vi "Draw Action Diagram.vi"(7 "Diagram Ref":refnum<vi>, 10 "Actions":T1) -> (2 "Action Diagram":picture)   [LabVIEW 2022 SP3, in "FlexBlocks Support.lvlib"]
uses:
  FlexBlocks Support.lvlib
  Action Selections.ctl
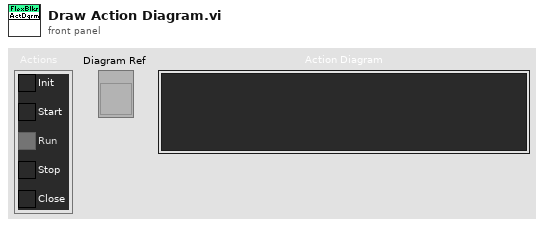
[diagram p1: front panel]
types:
  T1 = typedef "FlexBlocks Support.lvlib/Action Selections.ctl" = cluster{"Init":bool, "Start":bool, "Run":bool, "Stop":bool, "Close":bool}
  T2 = cluster{"left":i16, "top":i16, "right":i16, "bottom":i16}
  T3 = typedef "FlexBlocks Support.lvlib/Action Diagram Sizing.ctl" = cluster{"Start X":i32, "Node Spacing":i32, "Node Height":i32, "Node Center Offset":i32, "Terminus Spacing":i32, "Node Width":i32, "Total Width":i32, "Top":i32, "Inner Top":i32, "Outer Top":i32, "Line left":i32, "Line top":i32, "Line right":i32}
  T4 = cluster{"horizontal":enum16{"left", "center", "right"}, "vertical":enum16{"top", "center", "bottom"}}
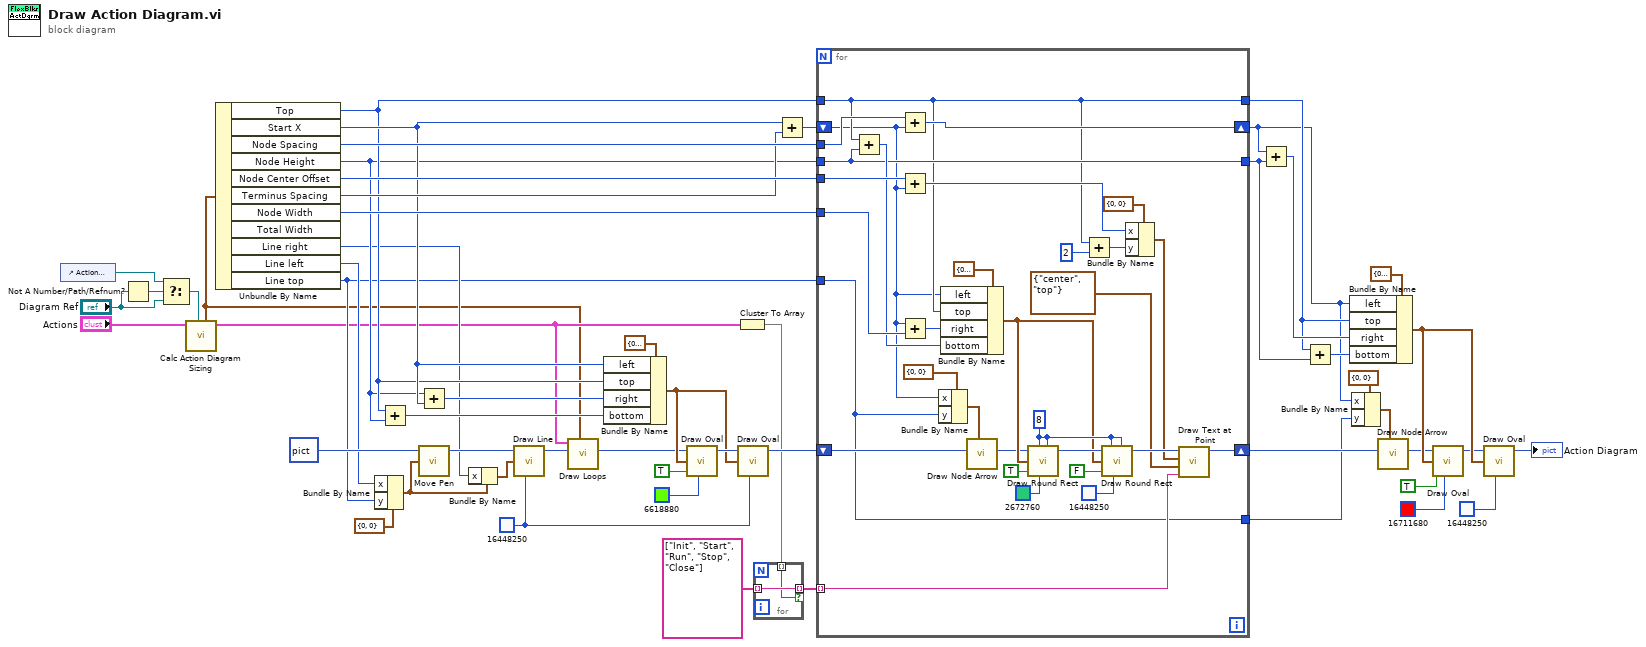
[diagram p0: block diagram]
diagram:
  w16 = u32 16448250 ("color(black)")
  n1 = control-ref of="Action Diagram"() -> (w25:refnum<vi>)
  n2 = Not A Number/Path/Refnum?(number/path/refnum="Diagram Ref") -> (NaN/Path/Refnum?=w26:bool)
  n3 = Select(t=w25, s=w26, f="Diagram Ref") -> (s? t:f=w23:refnum<vi>)
  n4 = call "Calc Action Diagram Sizing.vi"("Diagram Ref"=w23, "Actions In"="Actions") -> ("Actions"=w2:T1, "Action Diagram Sizing"=w1:T3)  [unwired: 8 in]
  n5 = Unbundle By Name(w1) -> ("Top"=w19:i32, "Start X"=w20:i32, "Node Spacing"=w36:i32, "Node Height"=w18:i32, "Node Center Offset"=w35:i32, "Terminus Spacing"=w32:i32, "Node Width"=w33:i32, "Line right"=w12:i32, "Line left"=w13:i32, "Line top"=w11:i32)  [unwired: 1 out]
  n6 = Bundle By Name(cluster=cluster{"x":i16, "y":i16} {"x"=0, "y"=0} ("new position"), "x"=w13, "y"=w11) -> (w15:cluster{"x":i16, "y":i16})
  n7 = Add(x=w19, y=w18) -> (x+y=w46:i32)
  n8 = Add(x=w18, y=w20) -> (x+y=w34:i32)
  n9 = call <vilib>:"Move Pen.vi"("new position"=w15, "picture"=picture data[5B] ("Action Diagram")) -> ("new picture"=w17:picture)  [unwired: 3 in]
  n10 = Bundle By Name(cluster=w15, "x"=w12) -> (w14:cluster{"x":i16, "y":i16})
  n11 = call <vilib>:"Draw Line.vi"("picture"=w17, "end point"=w14, "color(black)"=w16) -> ("new picture"=w4:picture)  [unwired: 6 in]
  n12 = call "Draw Loops.vi"("Action Diagram Sizing"=w1, "Action Diagram In"=w4, "Actions"=w2) -> ("Action Diagram"=w3:picture)  [unwired: 8 in]
  n13 = Bundle By Name(cluster=T2 {"left"=0, "top"=0, "right"=0, "bottom"=0} ("rect"), "left"=w20, "top"=w19, "right"=w34, "bottom"=w46) -> (w47:T2)
  n14 = call <vilib>:"Draw Oval.vi"("picture"=w3, "rect"=w47, "fill?(F)"=TRUE, "color(black)"=u32 6618880) -> ("new picture"=w49:picture)  [unwired: 5 in]
  n15 = Cluster To Array(cluster=w2) -> (array=w37:bool[])
  n16 = call <vilib>:"Draw Oval.vi"("picture"=w49, "rect"=w47, "color(black)"=w16) -> ("new picture"=w48:picture)  [unwired: 6 in]
  n17 = for {
    tunnel: string[] ["Init", "Start", "Run", "Stop", "Close"] -> [w56] mode=indexing
    tunnel: [w56] -> w53 mode=indexing if=w55
    tunnel: w37 -> [w55] mode=indexing
  }
  n18 = Add(x=w20, y=w32) -> (x+y=w31:i32)
  n19 = for {
    shift-right: [w79] -> w10
    shift-left: w48 -> [w61]
    tunnel: w53 -> [w78] mode=indexing
    tunnel: w19 -> [w63]
    tunnel: w36 -> [w66]
    tunnel: w18 -> [w64]
    tunnel: w35 -> [w71]
    shift-right: [w67] -> w6
    shift-left: w31 -> [w58]
    tunnel: w33 -> [w74]
    tunnel: [w64] -> w27
    tunnel: [w63] -> w28
    tunnel: w11 -> [w57]
    tunnel: [w57] -> w5
    w82 = i16 8 ("oval width")
    n20 = Add(x=w63, y=w64) -> (x+y=w65:i32)
    n21 = Add(x=w66, y=w58) -> (x+y=w67:i32)
    n22 = Add(x=w71, y=w58) -> (x+y=w70:i32)
    n23 = Add(x=w58, y=w74) -> (x+y=w75:i32)
    n24 = Bundle By Name(cluster=cluster{"x":i16, "y":i16} {"x"=0, "y"=0} ("Point"), "x"=w58, "y"=w57) -> (w59:cluster{"x":i16, "y":i16})
    n25 = Bundle By Name(cluster=T2 {"left"=0, "top"=0, "right"=0, "bottom"=0} ("rect"), "left"=w58, "top"=w63, "right"=w75, "bottom"=w65) -> (w81:T2)
    n26 = call "Draw Node Arrow.vi"("Point"=w59, "Action Diagram In"=w61) -> ("Action Diagram"=w62:picture)  [unwired: 9 in]
    n27 = call <vilib>:"Draw Round Rect.vi"("picture"=w62, "oval width"=w82, "rect"=w81, "fill?(F)"=TRUE, "color(black)"=u32 2672760, "oval height"=w82) -> ("new picture"=w86:picture)  [unwired: 3 in]
    n28 = Add(x=w63, y=2) -> (x+y=w69:i32)
    n29 = call <vilib>:"Draw Round Rect.vi"("picture"=w86, "oval width"=w82, "rect"=w81, "fill?(F)"=FALSE, "color(black)"=u32 16448250, "oval height"=w82) -> ("new picture"=w80:picture)  [unwired: 3 in]
    n30 = Bundle By Name(cluster=cluster{"x":i16, "y":i16} {"x"=0, "y"=0} ("origin"), "x"=w70, "y"=w69) -> (w72:cluster{"x":i16, "y":i16})
    n31 = call <vilib>:"Draw Text at Point.vi"("text"=w78, "alignment(left, top)"=T4 {"horizontal"=enum."center", "vertical"=enum."top"}, "origin"=w72, "picture"=w80) -> ("new picture"=w79:picture)  [unwired: 6 in, 1 out]
  }
  n32 = Add(x=w6, y=w27) -> (x+y=w30:i32)
  n33 = Add(x=w28, y=w27) -> (x+y=w29:i32)
  n34 = Bundle By Name(cluster=T2 {"left"=0, "top"=0, "right"=0, "bottom"=0} ("rect"), "left"=w6, "top"=w28, "right"=w30, "bottom"=w29) -> (w45:T2)
  n35 = Bundle By Name(cluster=cluster{"x":i16, "y":i16} {"x"=0, "y"=0} ("Point"), "x"=w6, "y"=w5) -> (w7:cluster{"x":i16, "y":i16})
  n36 = call "Draw Node Arrow.vi"("Point"=w7, "Action Diagram In"=w10) -> ("Action Diagram"=w9:picture)  [unwired: 9 in]
  n37 = call <vilib>:"Draw Oval.vi"("picture"=w9, "rect"=w45, "fill?(F)"=TRUE, "color(black)"=u32 16711680) -> ("new picture"=w43:picture)  [unwired: 5 in]
  n38 = call <vilib>:"Draw Oval.vi"("picture"=w43, "rect"=w45, "color(black)"=u32 16448250) -> ("new picture"=→"Action Diagram":picture)  [unwired: 6 in]
